vi "TH2829RUN.vi"(0 "仪器通讯端口":refnum<visa-resource-name>) -> (14 "VISA resource name out":refnum<visa-resource-name>, 15 "Turns Result":sgl[][](array[numeric]) format="%#_6f", 16 "Lx Result":sgl[][](array[numeric]) format="%#_6f", 17 "Lk Result":sgl[][](array[numeric]) format="%#_6f", 18 "DCR Result":sgl[][](array[numeric]) format="%#_6f")   [LabVIEW 2018]
panel:
  out "LED IrCompare Result":u8[][](array[numeric])
  out "LED VfCompare Result":u8[][](array[numeric])
  out "LED IrResult":sgl[][](array[numeric]) format="%#_6f"
  out "LED VfResult":sgl[][](array[numeric]) format="%#_6f"
  out "Bls Result":sgl[][](array[numeric]) format="%#_6f"
  out "总判断":u8
  out "PS Compare Result":u8[][](array[numeric])
  out "Balance Compare Result":u8[][](array[numeric])
  out "Z Compare Result":u8[][](array[numeric])
  out "Rs Compare Result":u8[][](array[numeric])
  out "LxQ Compare Result":u8[][](array[numeric])
  out "DCR Compare Result":u8[][](array[numeric])
  out "C Compare Result":u8[][](array[numeric])
  out "Lk Compare Result":u8[][](array[numeric])
  out "Lx Compare Result":u8[][](array[numeric])
  out "Turns Compare Result":u8[][](array[numeric])
  out "Polarity Result1":string[][](array[string])
  out "Polarity Result":u8[][](array[numeric])
  out "Zx Result":sgl[][](array[numeric]) format="%#_6f"
  out "ACR Result":sgl[][](array[numeric]) format="%#_6f"
  out "LxQ Result":sgl[][](array[numeric]) format="%#_6f"
  out "Cx Result":sgl[][](array[numeric]) format="%#_6f"
  out "Primary Sets":string
  out "head":string
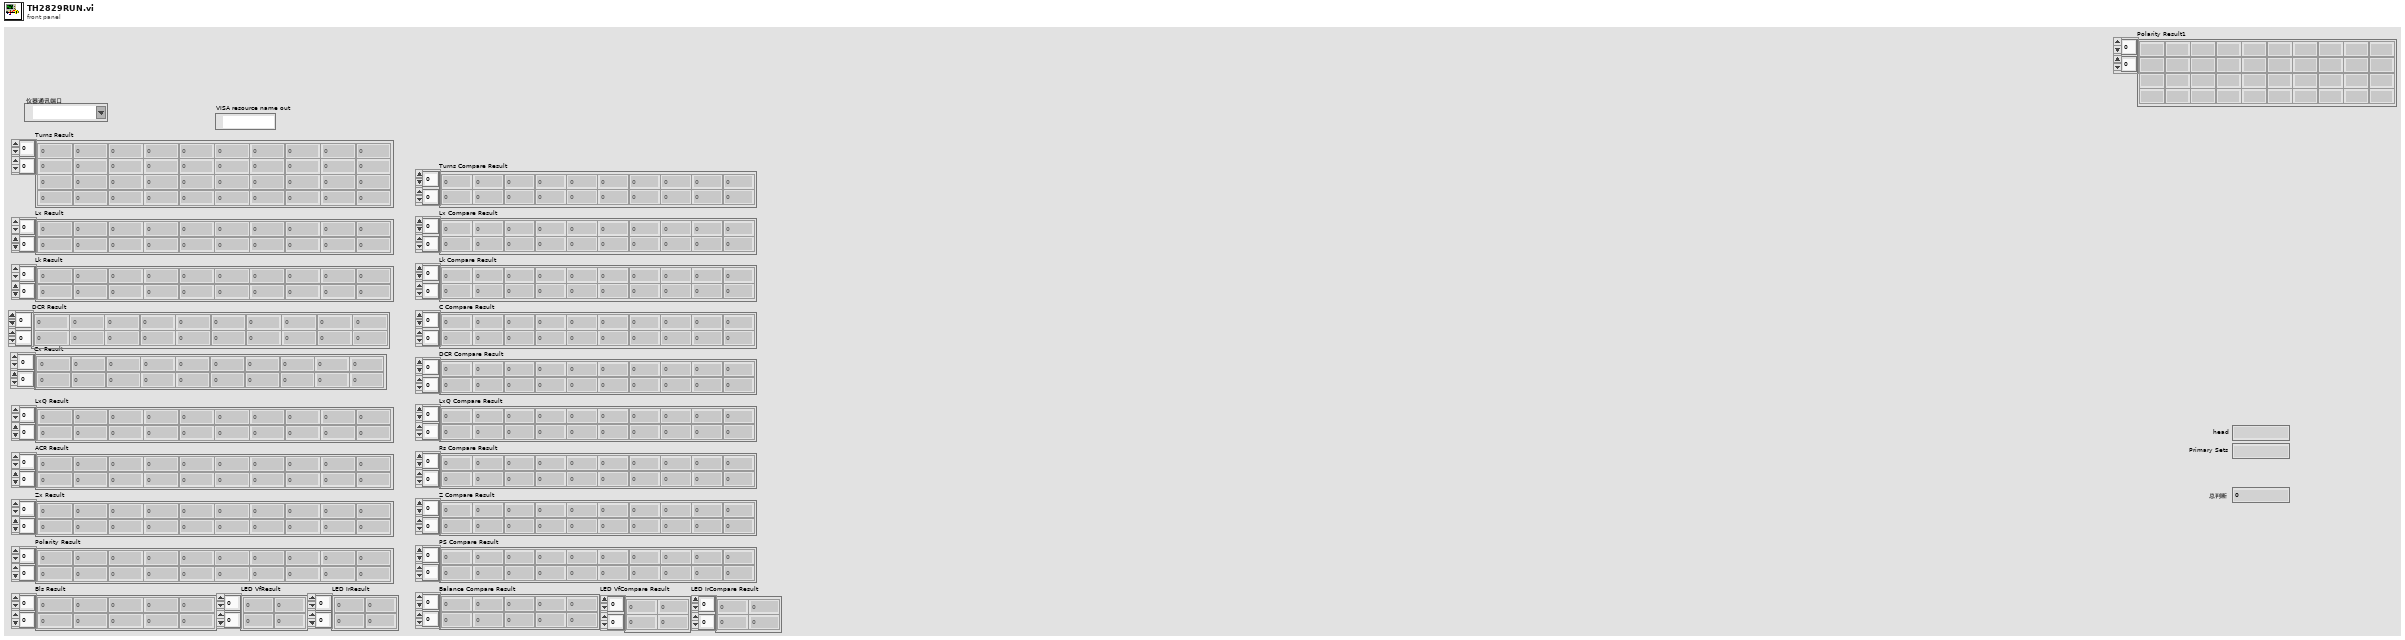
[diagram p1: front panel]
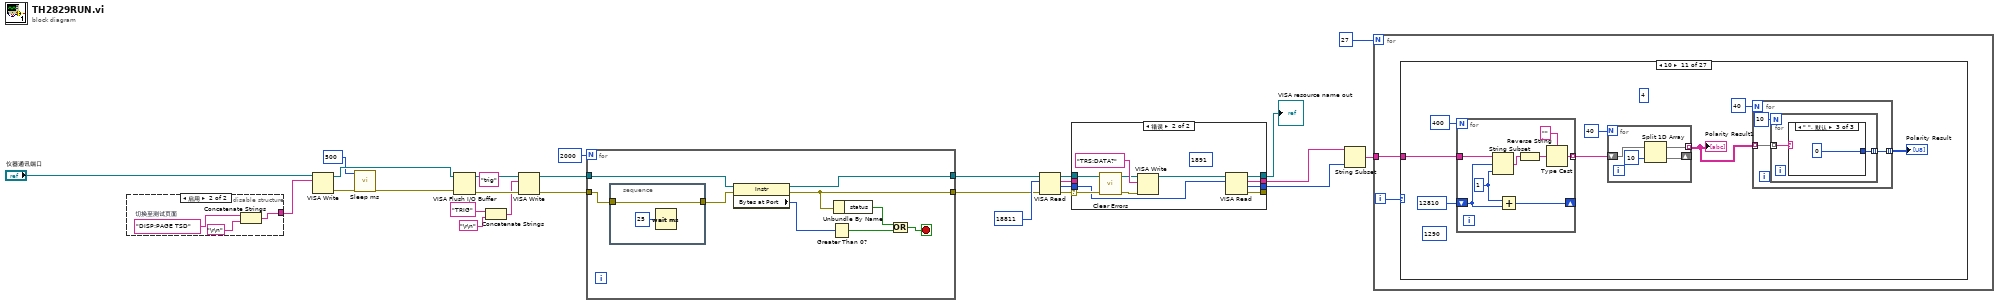
[diagram p0: block diagram]
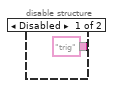
[diagram p2: hidden frame]
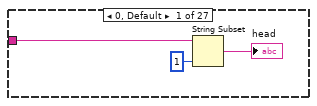
[diagram p3: hidden frame]
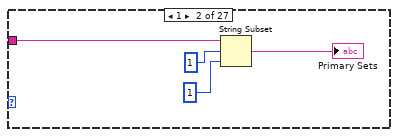
[diagram p4: hidden frame]
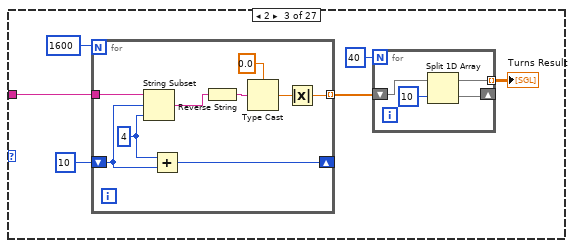
[diagram p5: hidden frame]
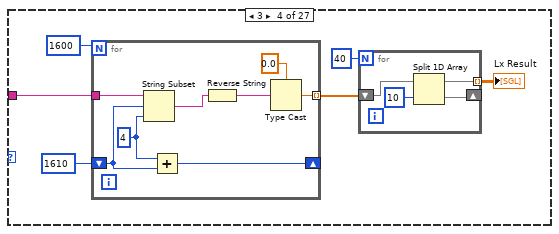
[diagram p6: hidden frame]
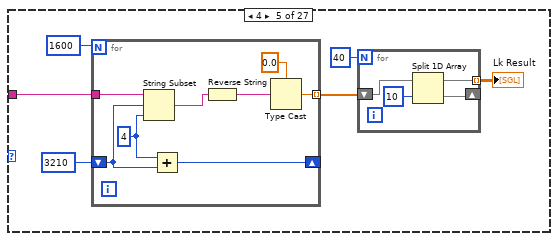
[diagram p7: hidden frame]
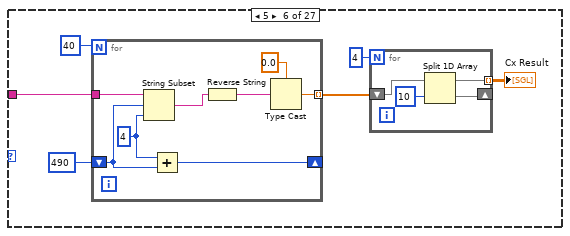
[diagram p8: hidden frame]
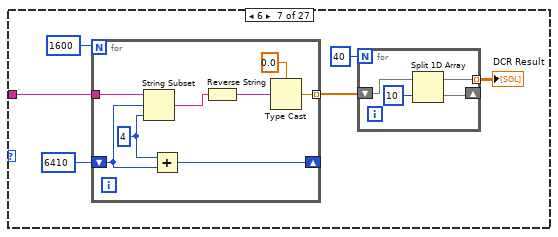
[diagram p9: hidden frame]
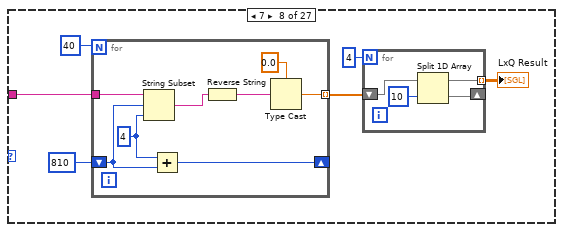
[diagram p10: hidden frame]
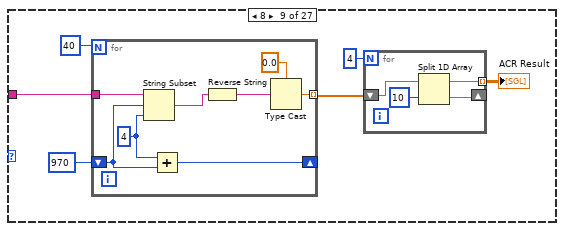
[diagram p11: hidden frame]
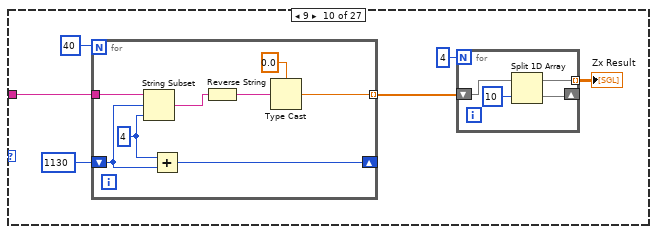
[diagram p12: hidden frame]
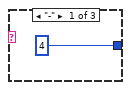
[diagram p13: hidden frame]
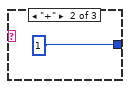
[diagram p14: hidden frame]
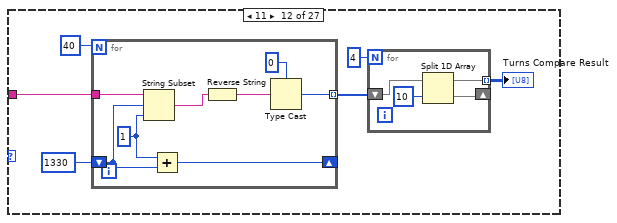
[diagram p15: hidden frame]
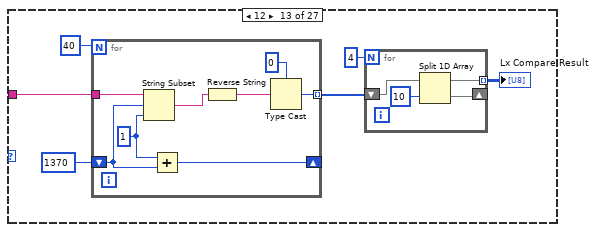
[diagram p16: hidden frame]
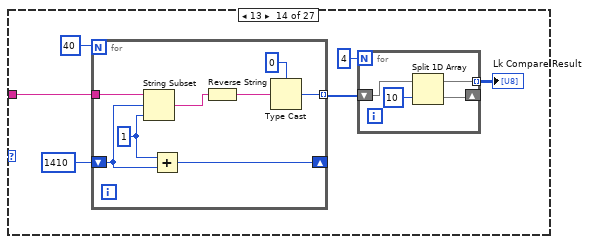
[diagram p17: hidden frame]
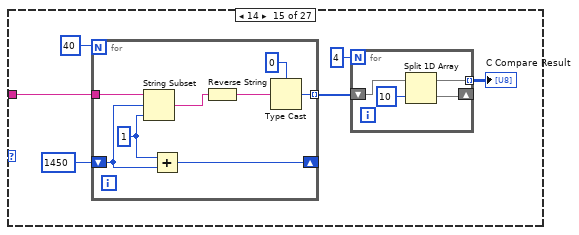
[diagram p18: hidden frame]
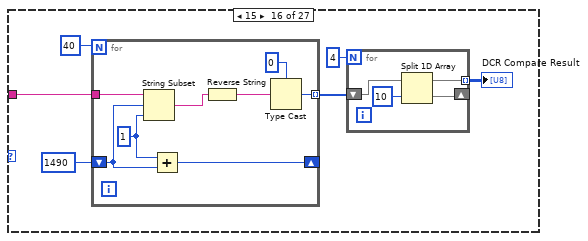
[diagram p19: hidden frame]
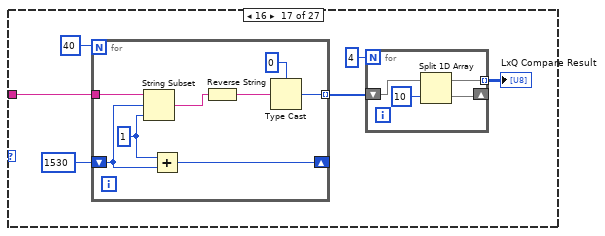
[diagram p20: hidden frame]
diagram:
  (unwired) "trig" ("write buffer")
  n1 = disable-structure shown="启用" {
    disable-tunnel: ["trig" ("write buffer") w28] -> w3
    frame Disabled {
    }
    frame Enabled {
      w29 = "DISP:PAGE TSD"  # 切换至测试页面
      n2 = Concatenate Strings(w29, "\r\n") -> (w28:string)
    }
  }
  n3 = VISA Write(VISA resource name="仪器通讯端口", write buffer=w3) -> (VISA resource name out=w4:refnum<visa-resource-name>, error out=w2:errorcluster)  [unwired: 1 in, 1 out]
  n4 = call "Sleep ms.vi"("error in (no error)"=w2, "等待时间（毫秒）"=u32 500) -> ("error out"=w5:errorcluster)  [unwired: 9 in]
  n5 = VISA Flush I/O Buffer(VISA resource name=w4, error in (no error)=w5) -> (VISA resource name out=w18:refnum<visa-resource-name>, error out=w17:errorcluster)  [unwired: 1 in]
  n6 = Concatenate Strings("TRIG" ("write buffer"), "\r\n") -> (w6:string)
  n7 = VISA Write(VISA resource name=w18, write buffer=w6, error in (no error)=w17) -> (VISA resource name out=w21:refnum<visa-resource-name>, error out=w10:errorcluster)  [unwired: 1 out]
  n8 = for {
    N: 2000 -> [_]
    tunnel: w21 -> [w39]
    tunnel: w10 -> [w31]
    tunnel: [w38] -> w19
    tunnel: [w35] -> w20
    stop <- w33 stop-if-true
    n9 = stacked-sequence {
      tunnel: [w41] -> w32
      tunnel: w31 -> [w41]
      frame #0 {
        n10 = Wait (ms)(milliseconds to wait=u32 25 ("等待时间（毫秒）")) -> ()  [unwired: 1 out]
      }
    }
    n11 = property class="Instr"(reference=w39, error in=w32) -> (reference out=w38:refnum<visa-resource-name>, error out=w35:errorcluster, "Bytes at Port"=w37:u32)
    n12 = Greater Than 0?(x=w37) -> (x > 0?=w36:bool)
    n13 = Unbundle By Name(w35) -> ("status"=w34:bool)
    n14 = Or(x=w34, y=w36) -> (x .or. y?=w33:bool)
  }
  n15 = VISA Read(VISA resource name=w19, byte count=u32 18811 ("字节总数"), error in (no error)=w20) -> (VISA resource name out=w24:refnum<visa-resource-name>, read buffer=w26:string, return count=w25:u32, error out=w23:errorcluster)
  n16 = case shown="错误" w23 {
    selector: w23 -> [w45 w52]
    tunnel: w24 -> [w44 w51]
    tunnel: [w44 w50] -> w12
    tunnel: [w45 w49] -> _
    tunnel: [w42 w48] -> w13
    tunnel: [w43 w47] -> w14
    tunnel: w25 -> [w43 w46]
    tunnel: w26 -> [w42 _]
    frame No Error {
    }
    frame Error {
      (unwired) u32 1891 ("字节总数")
      n17 = call <vilib>:"Clear Errors.vi"("error in (no error)"=w52) -> ("error out"=w53:errorcluster)  [unwired: 5 in, 1 out]
      n18 = VISA Write(VISA resource name=w51, write buffer="TRS:DATA?", error in (no error)=w53) -> (VISA resource name out=w55:refnum<visa-resource-name>)  [unwired: 2 out]
      n19 = VISA Read(VISA resource name=w55, byte count=w46) -> (VISA resource name out=w50:refnum<visa-resource-name>, read buffer=w48:string, return count=w47:u32, error out=w49:errorcluster)  [unwired: 1 in]
    }
  }
  "VISA resource name out" <- w12
  n20 = String Subset(string=w13, length (rest)=w14) -> (substring=w15:string)  [unwired: 1 in]
  n21 = for {
    N: 27 -> [_]
    tunnel: w15 -> [w56]
    i -> [w57]
    n22 = case shown="10" w57 {
      tunnel: w56 -> [w60 w64 w69 w88 w106 w124 w142 w160 w178 w196 w216 w242 w260 w278 w296 w314 w332 w350 w368 w386 w404 w421 w425 w443 w461 w479 w497]
      frame 0, Default {
        n23 = String Subset(string=w60, length (rest)=1 ("长度（剩余）")) -> (substring=→"head":string)  [unwired: 1 in]
      }
      frame 1 {
        n24 = String Subset ("截取字符串")(string=w64, offset (0)=1 ("长度（剩余）"), length (rest)=1 ("长度（剩余）")) -> (substring=→"Primary Sets":string)
      }
      frame 2 {
        n25 = for {
          N: 1600 -> [_]
          shift-right: [w79] -> _
          shift-left: 10 ("长度（剩余）") -> [w75]
          tunnel: w69 -> [w74]
          tunnel: [w71] -> w67 mode=indexing
          w76 = 4 ("长度（剩余）")
          n26 = String Subset(string=w74, offset (0)=w75, length (rest)=w76) -> (substring=w73:string)
          n27 = Add(x=w76, y=w75) -> (x+y=w79:i32)
          n28 = Reverse String(1:w73) -> (0:w78:string)
          n29 = Type Cast(type=sgl 0.0 ("长度（剩余）"), x=w78) -> (*(type *) &x=w72:sgl)
          n30 = Absolute Value(x=w72) -> (abs(x)=w71:sgl)
        }
        n31 = for {
          N: 40 -> [_]
          shift-right: [w82] -> _
          shift-left: w67 -> [w80]
          tunnel: [w81] -> w65 mode=indexing
          n32 = Split 1D Array(array=w80, index=10 ("索引")) -> (first subarray=w81:sgl[], second subarray=w82:sgl[])
        }
        "Turns Result" <- w65
      }
      frame 3 {
        n33 = for {
          N: 1600 -> [_]
          shift-right: [w97] -> _
          shift-left: 1610 ("长度（剩余）") -> [w93]
          tunnel: w88 -> [w92]
          tunnel: [w90] -> w86 mode=indexing
          w94 = 4 ("长度（剩余）")
          n34 = String Subset(string=w92, offset (0)=w93, length (rest)=w94) -> (substring=w91:string)
          n35 = Add(x=w94, y=w93) -> (x+y=w97:i32)
          n36 = Reverse String(1:w91) -> (0:w96:string)
          n37 = Type Cast(type=sgl 0.0 ("长度（剩余）"), x=w96) -> (*(type *) &x=w90:sgl)
        }
        n38 = for {
          N: 40 -> [_]
          shift-right: [w100] -> _
          shift-left: w86 -> [w98]
          tunnel: [w99] -> w84 mode=indexing
          n39 = Split 1D Array(array=w98, index=10 ("索引")) -> (first subarray=w99:sgl[], second subarray=w100:sgl[])
        }
        "Lx Result" <- w84
      }
      frame 4 {
        n40 = for {
          N: 1600 -> [_]
          shift-right: [w115] -> _
          shift-left: 3210 ("长度（剩余）") -> [w111]
          tunnel: w106 -> [w110]
          tunnel: [w108] -> w104 mode=indexing
          w112 = 4 ("长度（剩余）")
          n41 = String Subset(string=w110, offset (0)=w111, length (rest)=w112) -> (substring=w109:string)
          n42 = Add(x=w112, y=w111) -> (x+y=w115:i32)
          n43 = Reverse String(1:w109) -> (0:w114:string)
          n44 = Type Cast(type=sgl 0.0 ("长度（剩余）"), x=w114) -> (*(type *) &x=w108:sgl)
        }
        n45 = for {
          N: 40 -> [_]
          shift-right: [w118] -> _
          shift-left: w104 -> [w116]
          tunnel: [w117] -> w102 mode=indexing
          n46 = Split 1D Array(array=w116, index=10 ("索引")) -> (first subarray=w117:sgl[], second subarray=w118:sgl[])
        }
        "Lk Result" <- w102
      }
      frame 5 {
        n47 = for {
          N: 40 -> [_]
          shift-right: [w133] -> _
          shift-left: 490 ("长度（剩余）") -> [w129]
          tunnel: w124 -> [w128]
          tunnel: [w126] -> w122 mode=indexing
          w130 = 4 ("长度（剩余）")
          n48 = String Subset(string=w128, offset (0)=w129, length (rest)=w130) -> (substring=w127:string)
          n49 = Add(x=w130, y=w129) -> (x+y=w133:i32)
          n50 = Reverse String(1:w127) -> (0:w132:string)
          n51 = Type Cast(type=sgl 0.0 ("长度（剩余）"), x=w132) -> (*(type *) &x=w126:sgl)
        }
        n52 = for {
          N: 4 -> [_]
          shift-right: [w136] -> _
          shift-left: w122 -> [w134]
          tunnel: [w135] -> w120 mode=indexing
          n53 = Split 1D Array(array=w134, index=10 ("索引")) -> (first subarray=w135:sgl[], second subarray=w136:sgl[])
        }
        "Cx Result" <- w120
      }
      frame 6 {
        n54 = for {
          N: 1600 -> [_]
          shift-right: [w151] -> _
          shift-left: 6410 ("长度（剩余）") -> [w147]
          tunnel: w142 -> [w146]
          tunnel: [w144] -> w140 mode=indexing
          w148 = 4 ("长度（剩余）")
          n55 = String Subset(string=w146, offset (0)=w147, length (rest)=w148) -> (substring=w145:string)
          n56 = Add(x=w148, y=w147) -> (x+y=w151:i32)
          n57 = Reverse String(1:w145) -> (0:w150:string)
          n58 = Type Cast(type=sgl 0.0 ("长度（剩余）"), x=w150) -> (*(type *) &x=w144:sgl)
        }
        n59 = for {
          N: 40 -> [_]
          shift-right: [w154] -> _
          shift-left: w140 -> [w152]
          tunnel: [w153] -> w138 mode=indexing
          n60 = Split 1D Array(array=w152, index=10 ("索引")) -> (first subarray=w153:sgl[], second subarray=w154:sgl[])
        }
        "DCR Result" <- w138
      }
      frame 7 {
        n61 = for {
          N: 40 -> [_]
          shift-right: [w169] -> _
          shift-left: 810 ("长度（剩余）") -> [w165]
          tunnel: w160 -> [w164]
          tunnel: [w162] -> w158 mode=indexing
          w166 = 4 ("长度（剩余）")
          n62 = String Subset(string=w164, offset (0)=w165, length (rest)=w166) -> (substring=w163:string)
          n63 = Add(x=w166, y=w165) -> (x+y=w169:i32)
          n64 = Reverse String(1:w163) -> (0:w168:string)
          n65 = Type Cast(type=sgl 0.0 ("长度（剩余）"), x=w168) -> (*(type *) &x=w162:sgl)
        }
        n66 = for {
          N: 4 -> [_]
          shift-right: [w172] -> _
          shift-left: w158 -> [w170]
          tunnel: [w171] -> w156 mode=indexing
          n67 = Split 1D Array(array=w170, index=10 ("索引")) -> (first subarray=w171:sgl[], second subarray=w172:sgl[])
        }
        "LxQ Result" <- w156
      }
      frame 8 {
        n68 = for {
          N: 40 -> [_]
          shift-right: [w187] -> _
          shift-left: 970 ("长度（剩余）") -> [w183]
          tunnel: w178 -> [w182]
          tunnel: [w180] -> w176 mode=indexing
          w184 = 4 ("长度（剩余）")
          n69 = String Subset(string=w182, offset (0)=w183, length (rest)=w184) -> (substring=w181:string)
          n70 = Add(x=w184, y=w183) -> (x+y=w187:i32)
          n71 = Reverse String(1:w181) -> (0:w186:string)
          n72 = Type Cast(type=sgl 0.0 ("长度（剩余）"), x=w186) -> (*(type *) &x=w180:sgl)
        }
        n73 = for {
          N: 4 -> [_]
          shift-right: [w190] -> _
          shift-left: w176 -> [w188]
          tunnel: [w189] -> w174 mode=indexing
          n74 = Split 1D Array(array=w188, index=10 ("索引")) -> (first subarray=w189:sgl[], second subarray=w190:sgl[])
        }
        "ACR Result" <- w174
      }
      frame 9 {
        n75 = for {
          N: 40 -> [_]
          shift-right: [w205] -> _
          shift-left: 1130 ("长度（剩余）") -> [w201]
          tunnel: w196 -> [w200]
          tunnel: [w198] -> w194 mode=indexing
          w202 = 4 ("长度（剩余）")
          n76 = String Subset(string=w200, offset (0)=w201, length (rest)=w202) -> (substring=w199:string)
          n77 = Add(x=w202, y=w201) -> (x+y=w205:i32)
          n78 = Reverse String(1:w199) -> (0:w204:string)
          n79 = Type Cast(type=sgl 0.0 ("长度（剩余）"), x=w204) -> (*(type *) &x=w198:sgl)
        }
        n80 = for {
          N: 4 -> [_]
          shift-right: [w208] -> _
          shift-left: w194 -> [w206]
          tunnel: [w207] -> w192 mode=indexing
          n81 = Split 1D Array(array=w206, index=10 ("索引")) -> (first subarray=w207:sgl[], second subarray=w208:sgl[])
        }
        "Zx Result" <- w192
      }
      frame 10 {
        (unwired) 1290 ("长度（剩余）")
        (unwired) 4
        n82 = for {
          N: 400 -> [_]
          shift-right: [w233] -> _
          shift-left: 12810 ("长度（剩余）") -> [w230]
          tunnel: w216 -> [w229]
          tunnel: [w227] -> w211 mode=indexing
          w231 = 1 ("长度（剩余）")
          n83 = String Subset(string=w229, offset (0)=w230, length (rest)=w231) -> (substring=w228:string)
          n84 = Add(x=w231, y=w230) -> (x+y=w233:i32)
          n85 = Reverse String(1:w228) -> (0:w232:string)
          n86 = Type Cast(type="", x=w232) -> (*(type *) &x=w227:string)
        }
        n87 = for {
          N: 40 -> [_]
          shift-right: [w236] -> _
          shift-left: w211 -> [w234]
          tunnel: [w235] -> w210 mode=indexing
          n88 = Split 1D Array(array=w234, index=10 ("索引")) -> (first subarray=w235:string[], second subarray=w236:string[])
        }
        "Polarity Result1" <- w210
        n89 = for {
          N: 40 -> [_]
          tunnel: w210 -> [w219] mode=indexing
          tunnel: [w218] -> w212 mode=indexing
          n90 = for {
            N: 10 -> [_]
            tunnel: w219 -> [w222] mode=indexing
            tunnel: [w221] -> w218 mode=indexing
            n91 = case shown="\" \", 默认" w222 {
              tunnel: [u8 4 u8 1 u8 0] -> w221
              frame "-" {
              }
              frame "+" {
              }
              frame " ", Default {
              }
            }
          }
        }
        "Polarity Result" <- w212
      }
      frame 11 {
        n92 = for {
          N: 40 -> [_]
          shift-right: [w251] -> _
          shift-left: 1330 ("长度（剩余）") -> [w247]
          tunnel: w242 -> [w246]
          tunnel: [w244] -> w240 mode=indexing
          w248 = 1 ("长度（剩余）")
          n93 = String Subset ("截取字符串")(string=w246, offset (0)=w247, length (rest)=w248) -> (substring=w245:string)
          n94 = Add(x=w248, y=w247) -> (x+y=w251:i32)
          n95 = Reverse String(1:w245) -> (0:w250:string)
          n96 = Type Cast(type=u8 0 ("长度（剩余）"), x=w250) -> (*(type *) &x=w244:u8)
        }
        n97 = for {
          N: 4 -> [_]
          shift-right: [w254] -> _
          shift-left: w240 -> [w252]
          tunnel: [w253] -> w238 mode=indexing
          n98 = Split 1D Array(array=w252, index=10 ("索引")) -> (first subarray=w253:u8[], second subarray=w254:u8[])
        }
        "Turns Compare Result" <- w238
      }
      frame 12 {
        n99 = for {
          N: 40 -> [_]
          shift-right: [w269] -> _
          shift-left: 1370 ("长度（剩余）") -> [w265]
          tunnel: w260 -> [w264]
          tunnel: [w262] -> w258 mode=indexing
          w266 = 1 ("长度（剩余）")
          n100 = String Subset(string=w264, offset (0)=w265, length (rest)=w266) -> (substring=w263:string)
          n101 = Add(x=w266, y=w265) -> (x+y=w269:i32)
          n102 = Reverse String(1:w263) -> (0:w268:string)
          n103 = Type Cast(type=u8 0 ("长度（剩余）"), x=w268) -> (*(type *) &x=w262:u8)
        }
        n104 = for {
          N: 4 -> [_]
          shift-right: [w272] -> _
          shift-left: w258 -> [w270]
          tunnel: [w271] -> w256 mode=indexing
          n105 = Split 1D Array(array=w270, index=10 ("索引")) -> (first subarray=w271:u8[], second subarray=w272:u8[])
        }
        "Lx Compare Result" <- w256
      }
      frame 13 {
        n106 = for {
          N: 40 -> [_]
          shift-right: [w287] -> _
          shift-left: 1410 ("长度（剩余）") -> [w283]
          tunnel: w278 -> [w282]
          tunnel: [w280] -> w276 mode=indexing
          w284 = 1 ("长度（剩余）")
          n107 = String Subset(string=w282, offset (0)=w283, length (rest)=w284) -> (substring=w281:string)
          n108 = Add(x=w284, y=w283) -> (x+y=w287:i32)
          n109 = Reverse String(1:w281) -> (0:w286:string)
          n110 = Type Cast(type=u8 0 ("长度（剩余）"), x=w286) -> (*(type *) &x=w280:u8)
        }
        n111 = for {
          N: 4 -> [_]
          shift-right: [w290] -> _
          shift-left: w276 -> [w288]
          tunnel: [w289] -> w274 mode=indexing
          n112 = Split 1D Array(array=w288, index=10 ("索引")) -> (first subarray=w289:u8[], second subarray=w290:u8[])
        }
        "Lk Compare Result" <- w274
      }
      frame 14 {
        n113 = for {
          N: 40 -> [_]
          shift-right: [w305] -> _
          shift-left: 1450 ("长度（剩余）") -> [w301]
          tunnel: w296 -> [w300]
          tunnel: [w298] -> w294 mode=indexing
          w302 = 1 ("长度（剩余）")
          n114 = String Subset(string=w300, offset (0)=w301, length (rest)=w302) -> (substring=w299:string)
          n115 = Add(x=w302, y=w301) -> (x+y=w305:i32)
          n116 = Reverse String(1:w299) -> (0:w304:string)
          n117 = Type Cast(type=u8 0 ("长度（剩余）"), x=w304) -> (*(type *) &x=w298:u8)
        }
        n118 = for {
          N: 4 -> [_]
          shift-right: [w308] -> _
          shift-left: w294 -> [w306]
          tunnel: [w307] -> w292 mode=indexing
          n119 = Split 1D Array(array=w306, index=10 ("索引")) -> (first subarray=w307:u8[], second subarray=w308:u8[])
        }
        "C Compare Result" <- w292
      }
      frame 15 {
        n120 = for {
          N: 40 -> [_]
          shift-right: [w323] -> _
          shift-left: 1490 ("长度（剩余）") -> [w319]
          tunnel: w314 -> [w318]
          tunnel: [w316] -> w312 mode=indexing
          w320 = 1 ("长度（剩余）")
          n121 = String Subset(string=w318, offset (0)=w319, length (rest)=w320) -> (substring=w317:string)
          n122 = Add(x=w320, y=w319) -> (x+y=w323:i32)
          n123 = Reverse String(1:w317) -> (0:w322:string)
          n124 = Type Cast(type=u8 0 ("长度（剩余）"), x=w322) -> (*(type *) &x=w316:u8)
        }
        n125 = for {
          N: 4 -> [_]
          shift-right: [w326] -> _
          shift-left: w312 -> [w324]
          tunnel: [w325] -> w310 mode=indexing
          n126 = Split 1D Array(array=w324, index=10 ("索引")) -> (first subarray=w325:u8[], second subarray=w326:u8[])
        }
        "DCR Compare Result" <- w310
      }
      frame 16 {
        n127 = for {
          N: 40 -> [_]
          shift-right: [w341] -> _
          shift-left: 1530 ("长度（剩余）") -> [w337]
          tunnel: w332 -> [w336]
          tunnel: [w334] -> w330 mode=indexing
          w338 = 1 ("长度（剩余）")
          n128 = String Subset(string=w336, offset (0)=w337, length (rest)=w338) -> (substring=w335:string)
          n129 = Add(x=w338, y=w337) -> (x+y=w341:i32)
          n130 = Reverse String(1:w335) -> (0:w340:string)
          n131 = Type Cast(type=u8 0 ("长度（剩余）"), x=w340) -> (*(type *) &x=w334:u8)
        }
        n132 = for {
          N: 4 -> [_]
          shift-right: [w344] -> _
          shift-left: w330 -> [w342]
          tunnel: [w343] -> w328 mode=indexing
          n133 = Split 1D Array(array=w342, index=10 ("索引")) -> (first subarray=w343:u8[], second subarray=w344:u8[])
        }
        "LxQ Compare Result" <- w328
      }
      frame 17 {
        n134 = for {
          N: 40 -> [_]
          shift-right: [w359] -> _
          shift-left: 1570 ("长度（剩余）") -> [w353]
          tunnel: w350 -> [w354]
          tunnel: [w355] -> w348 mode=indexing
          w352 = 1 ("长度（剩余）")
          n135 = String Subset(string=w354, offset (0)=w353, length (rest)=w352) -> (substring=w356:string)
          n136 = Add(x=w352, y=w353) -> (x+y=w359:i32)
          n137 = Reverse String(1:w356) -> (0:w358:string)
          n138 = Type Cast(type=u8 0 ("长度（剩余）"), x=w358) -> (*(type *) &x=w355:u8)
        }
        n139 = for {
          N: 4 -> [_]
          shift-right: [w362] -> _
          shift-left: w348 -> [w360]
          tunnel: [w361] -> w346 mode=indexing
          n140 = Split 1D Array(array=w360, index=10 ("索引")) -> (first subarray=w361:u8[], second subarray=w362:u8[])
        }
        "Rs Compare Result" <- w346
      }
      frame 18 {
        n141 = for {
          N: 40 -> [_]
          shift-right: [w377] -> _
          shift-left: 1610 ("长度（剩余）") -> [w371]
          tunnel: w368 -> [w372]
          tunnel: [w373] -> w366 mode=indexing
          w370 = 1 ("长度（剩余）")
          n142 = Add(x=w370, y=w371) -> (x+y=w377:i32)
          n143 = String Subset(string=w372, offset (0)=w371, length (rest)=w370) -> (substring=w374:string)
          n144 = Reverse String(1:w374) -> (0:w376:string)
          n145 = Type Cast(type=u8 0 ("长度（剩余）"), x=w376) -> (*(type *) &x=w373:u8)
        }
        n146 = for {
          N: 4 -> [_]
          shift-right: [w380] -> _
          shift-left: w366 -> [w378]
          tunnel: [w379] -> w364 mode=indexing
          n147 = Split 1D Array(array=w378, index=10 ("索引")) -> (first subarray=w379:u8[], second subarray=w380:u8[])
        }
        "Z Compare Result" <- w364
      }
      frame 19 {
        n148 = for {
          N: 40 -> [_]
          shift-right: [w395] -> _
          shift-left: 1650 ("长度（剩余）") -> [w390]
          tunnel: w386 -> [w391]
          tunnel: [w392] -> w384 mode=indexing
          w389 = 1 ("长度（剩余）")
          n149 = String Subset(string=w391, offset (0)=w390, length (rest)=w389) -> (substring=w393:string)
          n150 = Add(x=w389, y=w390) -> (x+y=w395:i32)
          n151 = Reverse String(1:w393) -> (0:w394:string)
          n152 = Type Cast(type=u8 0 ("长度（剩余）"), x=w394) -> (*(type *) &x=w392:u8)
        }
        n153 = for {
          N: 4 -> [_]
          shift-right: [w398] -> _
          shift-left: w384 -> [w396]
          tunnel: [w397] -> w382 mode=indexing
          n154 = Split 1D Array(array=w396, index=10 ("索引")) -> (first subarray=w397:u8[], second subarray=w398:u8[])
        }
        "Balance Compare Result" <- w382
      }
      frame 20 {
        n155 = for {
          N: 40 -> [_]
          shift-right: [w413] -> _
          shift-left: 1690 ("长度（剩余）") -> [w408]
          tunnel: w404 -> [w409]
          tunnel: [w410] -> w402 mode=indexing
          w407 = 1 ("长度（剩余）")
          n156 = String Subset(string=w409, offset (0)=w408, length (rest)=w407) -> (substring=w411:string)
          n157 = Add(x=w407, y=w408) -> (x+y=w413:i32)
          n158 = Reverse String(1:w411) -> (0:w412:string)
          n159 = Type Cast(type=u8 0 ("长度（剩余）"), x=w412) -> (*(type *) &x=w410:u8)
        }
        n160 = for {
          N: 4 -> [_]
          shift-right: [w416] -> _
          shift-left: w402 -> [w414]
          tunnel: [w415] -> w400 mode=indexing
          n161 = Split 1D Array(array=w414, index=10 ("索引")) -> (first subarray=w415:u8[], second subarray=w416:u8[])
        }
        "PS Compare Result" <- w400
      }
      frame 21 {
        n162 = String Subset(string=w421, offset (0)=1730 ("长度（剩余）"), length (rest)=1 ("长度（剩余）")) -> (substring=w424:string)
        n163 = Reverse String(1:w424) -> (0:w422:string)
        n164 = Type Cast(type=u8 0 ("长度（剩余）"), x=w422) -> (*(type *) &x=→"总判断":u8)
      }
      frame 22 {
        n165 = for {
          N: 20 -> [_]
          shift-right: [w438] -> _
          shift-left: 1731 ("长度（剩余）") -> [w434]
          tunnel: w425 -> [w433]
          tunnel: [w431] -> w428 mode=indexing
          w435 = 4 ("长度（剩余）")
          n166 = String Subset(string=w433, offset (0)=w434, length (rest)=w435) -> (substring=w432:string)
          n167 = Add(x=w435, y=w434) -> (x+y=w438:i32)
          n168 = Reverse String(1:w432) -> (0:w437:string)
          n169 = Type Cast(type=sgl 0.0 ("长度（剩余）"), x=w437) -> (*(type *) &x=w431:sgl)
        }
        n170 = for {
          N: 4 -> [_]
          shift-right: [w441] -> _
          shift-left: w428 -> [w439]
          tunnel: [w440] -> w426 mode=indexing
          n171 = Split 1D Array(array=w439, index=5 ("索引")) -> (first subarray=w440:sgl[], second subarray=w441:sgl[])
        }
        "Bls Result" <- w426
      }
      frame 23 {
        n172 = for {
          N: 8 -> [_]
          shift-right: [w456] -> _
          shift-left: 1811 ("长度（剩余）") -> [w452]
          tunnel: w443 -> [w451]
          tunnel: [w449] -> w445 mode=indexing
          w453 = 4 ("长度（剩余）")
          n173 = String Subset(string=w451, offset (0)=w452, length (rest)=w453) -> (substring=w450:string)
          n174 = Add(x=w453, y=w452) -> (x+y=w456:i32)
          n175 = Reverse String(1:w450) -> (0:w455:string)
          n176 = Type Cast(type=sgl 0.0 ("长度（剩余）"), x=w455) -> (*(type *) &x=w449:sgl)
        }
        n177 = for {
          N: 4 -> [_]
          shift-right: [w459] -> _
          shift-left: w445 -> [w457]
          tunnel: [w458] -> w448 mode=indexing
          n178 = Split 1D Array(array=w457, index=2 ("索引")) -> (first subarray=w458:sgl[], second subarray=w459:sgl[])
        }
        "LED VfResult" <- w448
      }
      frame 24 {
        n179 = for {
          N: 8 -> [_]
          shift-right: [w474] -> _
          shift-left: 1843 ("长度（剩余）") -> [w470]
          tunnel: w461 -> [w469]
          tunnel: [w467] -> w463 mode=indexing
          w471 = 4 ("长度（剩余）")
          n180 = String Subset(string=w469, offset (0)=w470, length (rest)=w471) -> (substring=w468:string)
          n181 = Add(x=w471, y=w470) -> (x+y=w474:i32)
          n182 = Reverse String(1:w468) -> (0:w473:string)
          n183 = Type Cast(type=sgl 0.0 ("长度（剩余）"), x=w473) -> (*(type *) &x=w467:sgl)
        }
        n184 = for {
          N: 4 -> [_]
          shift-right: [w477] -> _
          shift-left: w463 -> [w475]
          tunnel: [w476] -> w466 mode=indexing
          n185 = Split 1D Array(array=w475, index=2 ("索引")) -> (first subarray=w476:sgl[], second subarray=w477:sgl[])
        }
        "LED IrResult" <- w466
      }
      frame 25 {
        n186 = for {
          N: 8 -> [_]
          shift-right: [w492] -> _
          shift-left: 1875 ("长度（剩余）") -> [w487]
          tunnel: w479 -> [w488]
          tunnel: [w489] -> w481 mode=indexing
          w486 = 1 ("长度（剩余）")
          n187 = String Subset(string=w488, offset (0)=w487, length (rest)=w486) -> (substring=w490:string)
          n188 = Add(x=w486, y=w487) -> (x+y=w492:i32)
          n189 = Reverse String(1:w490) -> (0:w491:string)
          n190 = Type Cast(type=u8 0 ("长度（剩余）"), x=w491) -> (*(type *) &x=w489:u8)
        }
        n191 = for {
          N: 4 -> [_]
          shift-right: [w495] -> _
          shift-left: w481 -> [w493]
          tunnel: [w494] -> w484 mode=indexing
          n192 = Split 1D Array(array=w493, index=2 ("索引")) -> (first subarray=w494:u8[], second subarray=w495:u8[])
        }
        "LED VfCompare Result" <- w484
      }
      frame 26 {
        n193 = for {
          N: 8 -> [_]
          shift-right: [w510] -> _
          shift-left: 1883 ("长度（剩余）") -> [w505]
          tunnel: w497 -> [w506]
          tunnel: [w507] -> w499 mode=indexing
          w504 = 1 ("长度（剩余）")
          n194 = String Subset(string=w506, offset (0)=w505, length (rest)=w504) -> (substring=w508:string)
          n195 = Add(x=w504, y=w505) -> (x+y=w510:i32)
          n196 = Reverse String(1:w508) -> (0:w509:string)
          n197 = Type Cast(type=u8 0 ("长度（剩余）"), x=w509) -> (*(type *) &x=w507:u8)
        }
        n198 = for {
          N: 4 -> [_]
          shift-right: [w513] -> _
          shift-left: w499 -> [w511]
          tunnel: [w512] -> w502 mode=indexing
          n199 = Split 1D Array(array=w511, index=2 ("索引")) -> (first subarray=w512:u8[], second subarray=w513:u8[])
        }
        "LED IrCompare Result" <- w502
      }
    }
  }
